vi "wdt_absolutet0.vi"() -> ()   [LabVIEW 2019]
panel:
  out "Error Out":errorcluster
  in  "TDMS File":path=path "C:/Python/projects/nitdms/tests/tdms_files/wdt_absolutet0.tdms"
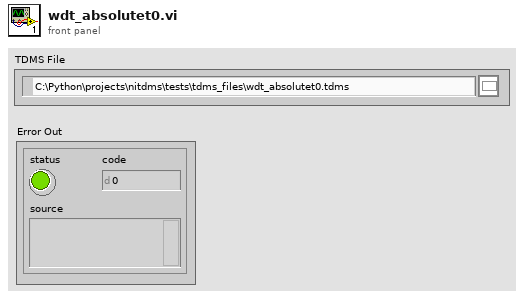
[diagram p1: front panel]
types:
  T1 = enum16{"open", "open or create", "create or replace", "create", "open (read-only)"}
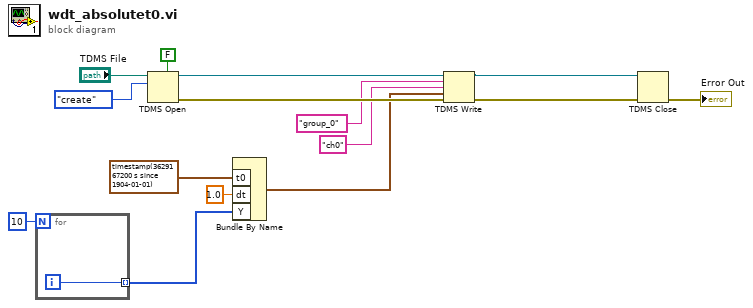
[diagram p0: block diagram]
diagram:
  n1 = for {
    N: 10 -> [_]
    tunnel: [w16] -> w5 mode=indexing
    i -> [w16]
  }
  n2 = TDMS Open(5:FALSE ("create index file? (T)"), 10:T1."create" ("operation (0:open)"), 11:"TDMS File") -> (0:w12:errorcluster, 3:w11:refnum<k34>)  [unwired: 4 in]
  n3 = Bundle By Name("t0"=timestamp(3629167200 s since 1904-01-01), "dt"=1.0, "Y"=w5) -> (w3:waveform(i32))  [unwired: 1 in]
  n4 = TDMS Write(0:w11, 5:"group_0" ("name"), 7:"ch0" ("name"), 9:w3, 11:w12) -> (4:w1:refnum<k34>, 15:w2:errorcluster)  [unwired: 1 in, 2 out]
  n5 = TDMS Close(8:w2, 11:w1) -> (0:→"Error Out":errorcluster)  [unwired: 1 out]
